vi "File Name Generator.vi"(1 "time string":string, 2 "date string":string, 3 "FileName":string="data") -> (0 "File Name":string)   [LabVIEW 2018]
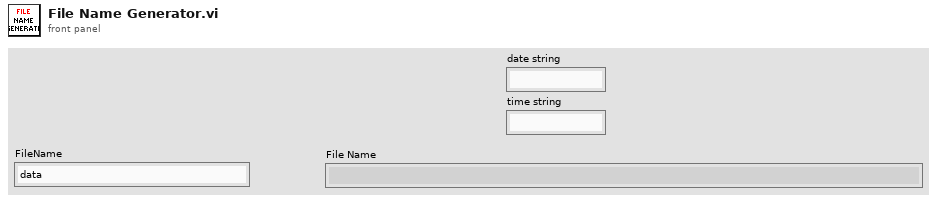
[diagram p1: front panel]
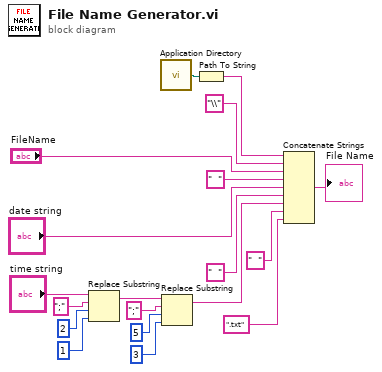
[diagram p0: block diagram]
diagram:
  n1 = Replace Substring(2:1 ("length (len. of substring)"), 3:2 ("offset (0)"), 4:";" ("substring (\"\")"), 5:"time string") -> (1:w9:string)  [unwired: 1 out]
  n2 = call <vilib>:"Application Directory.vi"() -> ("Application Directory"=w17:path)
  n3 = Replace Substring(2:3 ("length (len. of substring)"), 3:5 ("offset (0)"), 4:";" ("substring (\"\")"), 5:w9) -> (1:w3:string)  [unwired: 1 out]
  n4 = Path To String(path=w17) -> (string=w18:string)
  n5 = Concatenate Strings(w18, "\\" ("string"), "FileName", "  " ("string"), "date string", "  " ("string"), w3, "  " ("string"), ".txt" ("string")) -> (→"File Name":string)
